vi "Bit Masking.vi"() -> ()   [LabVIEW 2016]
panel:
  in  "Transmit?":bool
  out "Shifted Filter":u16 format="%016b"
  out "Final Address":u16 format="%04x"
  in  "Subaddress":u16 format="%0d"
  in  "RT Address":u16 format="%0d"
  in  "Bits to Check":i32=5
  out "Odd Parity Added":u16 format="%016b"
  in  "No Parity":u16 format="%016b"
  out "Shifted Register Value":u16 format="%016b"
  in  "Bit Offset":i32=15
  in  "Bit Count":i32=32
  out "Bit Mask":u16[](array[numeric]) format="%016b"
  out "Final Value":u16 format="%016b"
  in  "Register Value":u16 format="%016b"
  in  "Mask":u16 format="%016b"
  in  "Target Value":u16 format="%016b"
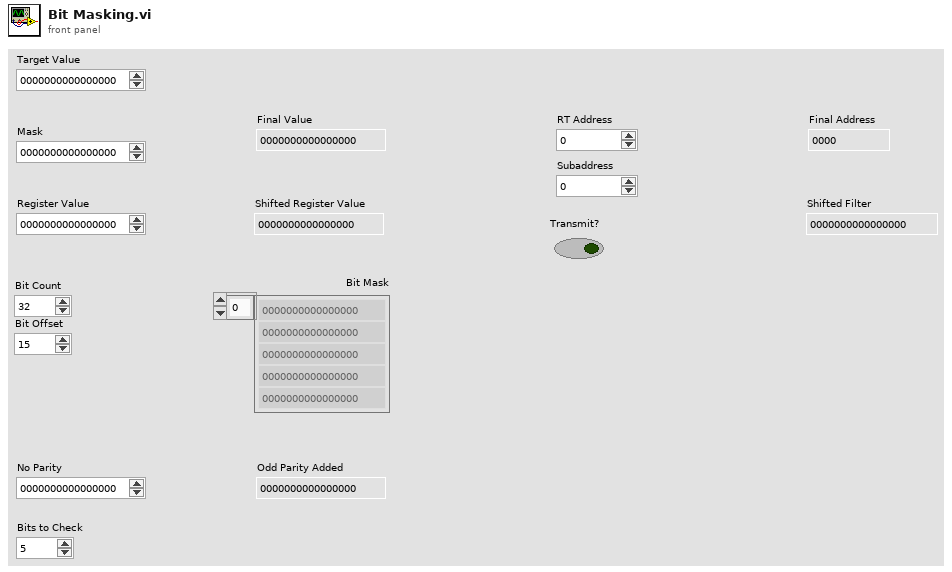
[diagram p1: front panel]
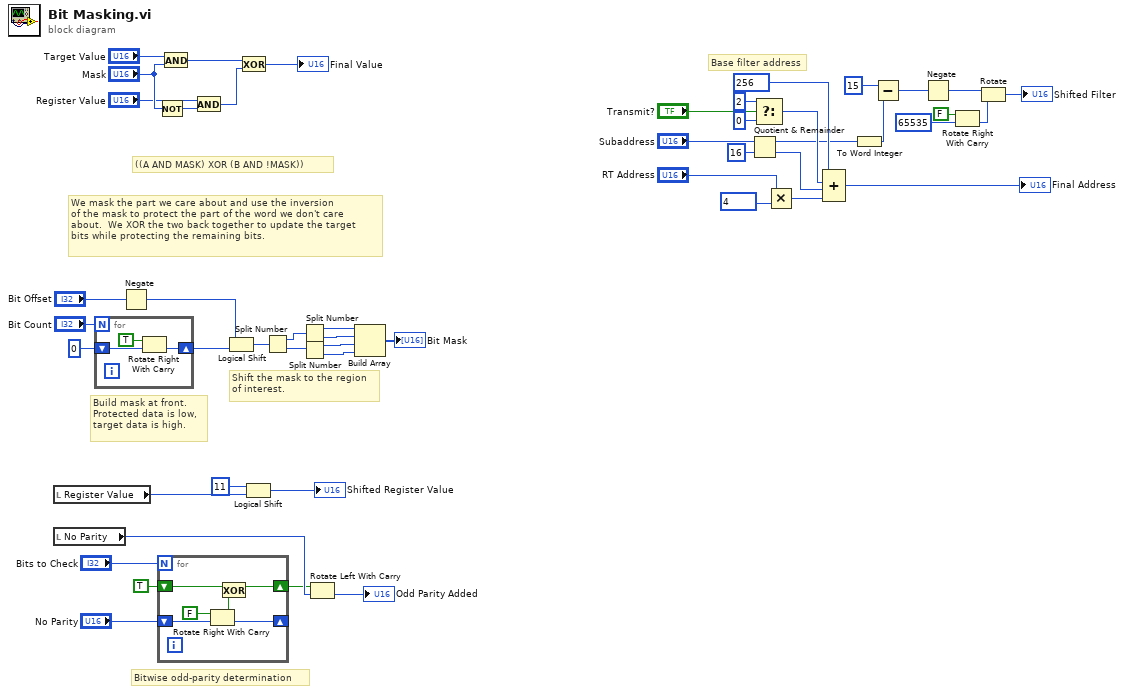
[diagram p0: block diagram]
diagram:
  # "Base filter address"
  # "Bitwise odd-parity determination"
  # "Shift the mask to the region\nof interest."
  # "Build mask at front.\nProtected data is low,\ntarget data is high."
  # "We mask the part we care about and use the inversion\nof the mask to protect the part of the word we don't care\nabout.  We XOR the two back together to update the target\nbits while protecting the remaining bits."
  # "((A AND MASK) XOR (B AND !MASK))"
  n1 = local read "Register Value"() -> (w29:u16)
  n2 = local read "No Parity"() -> (w24:u16)
  n3 = for {
    N: "Bit Count" -> [_]
    shift-right: [w52] -> w42
    shift-left: u64 0 -> [w53]
    n4 = Rotate Right With Carry(2:w53, 3:TRUE ("carry")) -> (0:w52:u64)  [unwired: 1 out]
  }
  n5 = Negate(x="Bit Offset") -> (-x=w31:i32)
  n6 = Not(x="Mask") -> (.not. x?=w46:u16)
  n7 = for {
    N: "Bits to Check" -> [_]
    shift-right: [w58] -> w23
    shift-left: TRUE -> [w59]
    shift-right: [w56] -> _
    shift-left: "No Parity" -> [w57]
    n8 = Rotate Right With Carry(2:w57, 3:FALSE ("carry")) -> (0:w56:u16, 1:w54:bool)
    n9 = Exclusive Or(1:w54, 2:w59) -> (0:w58:bool)
  }
  n10 = And(x="Target Value", y="Mask") -> (x .and. y?=w49:u16)
  n11 = And(x="Register Value", y=w46) -> (x .and. y?=w44:u16)
  n12 = Logical Shift(y=w31, x=w42) -> (x << y=w35:u64)
  n13 = Exclusive Or(1:w44, 2:w49) -> (0:→"Final Value":u16)
  n14 = Logical Shift(y=i16 11, x=w29) -> (x << y=→"Shifted Register Value":u16)
  n15 = Split Number(x=w35) -> (hi(x)=w36:u32, lo(x)=w41:u32)
  n16 = Split Number(x=w36) -> (hi(x)=w40:u16, lo(x)=w39:u16)
  n17 = Split Number(x=w41) -> (hi(x)=w38:u16, lo(x)=w37:u16)
  n18 = Rotate Left With Carry(2:w24, 3:w23) -> (0:→"Odd Parity Added":u16)  [unwired: 1 out]
  n19 = Build Array(w40, w39, w38, w37) -> (→"Bit Mask":u16[])
  n20 = Quotient & Remainder(x="Subaddress", y=u16 16) -> (x-y*floor(x/y)=w9:u16, floor(x/y)=w13:u16)
  n21 = Select(t=u16 2 ("y"), s="Transmit?", f=u16 0 ("y")) -> (s? t:f=w12:u16)
  n22 = Multiply(x="RT Address", y=u16 4) -> (x*y=w14:u16)
  n23 = Compound Arithmetic op=ADD(u16 256, w12, w13, w14) -> (→"Final Address":u16)
  n24 = To Word Integer(number=w9) -> (16bit integer=w2:i16)
  n25 = Subtract(x=i16 15 ("y"), y=w2) -> (x-y=w4:i16)
  n26 = Negate(x=w4) -> (-x=w1:i16)
  n27 = Rotate Right With Carry(2:u16 65535, 3:FALSE) -> (0:w5:u16)  [unwired: 1 out]
  n28 = Rotate(1:w5, 2:w1) -> (0:→"Shifted Filter":u16)
